vi "rewindDir_printDirectory.vi"(8 "Error In":errorcluster, 10 "nested level":u8, 11 "file":refnum<class "File.lvclass">) -> (0 "Error Out":errorcluster)   [LabVIEW 2014, in "LabVIEW Universal Transcriptor SD Card Library.lvlib"]
uses:
  LabVIEW Universal Transcriptor SD Card Library.lvlib
  File.lvclass
  File.lvclass/File.ctl
  File Class/Get If Rewind This Directory.vi
  <vilib>/Utility/file.llb/Application Directory.vi
  open.vi
  <vilib>/LabVIEW Universal Transcriptor/LabVIEW to Arduino Transcriptor/Transcriptors/System API/Serial println string.vi
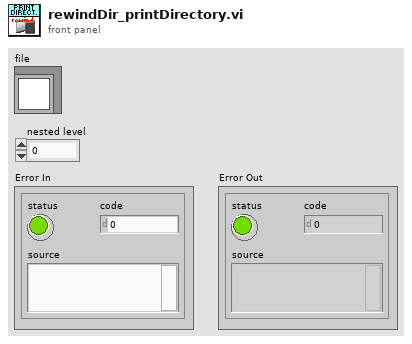
[diagram p1: front panel]
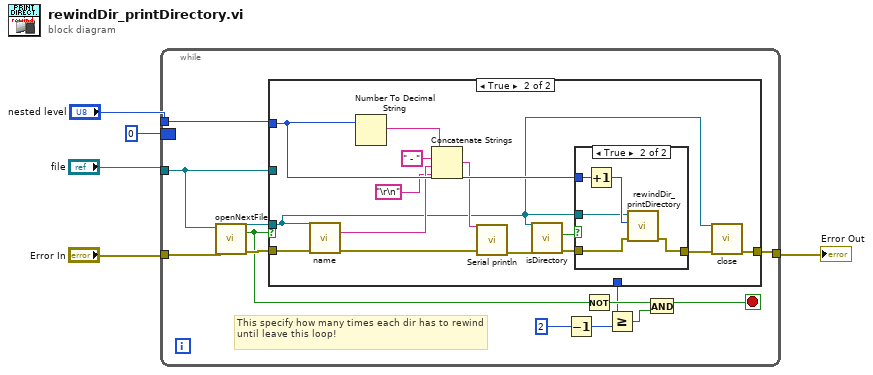
[diagram p0: block diagram]
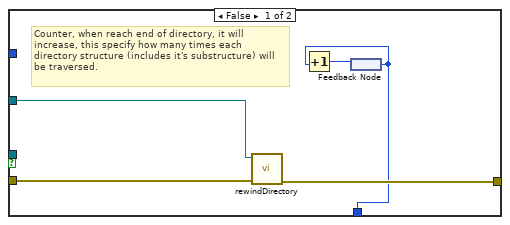
[diagram p2: hidden frame]
diagram:
  n1 = while {
    tunnel: "nested level" -> [w15]
    tunnel: "Error In" -> [w9]
    tunnel: [w16] -> w2
    tunnel: "file" -> [w8]
    border: 0 ("y") -> [_]
    stop <- w12 stop-if-true
    # "This specify how many times each dir has to rewind until leave this loop!"
    n2 = call "openNextFile.vi"("error in (no error)"=w9, "File in"=w8) -> ("error out"=w17:errorcluster, "success?"=w13:bool, "File out"=w18:refnum<class "File.lvclass">)  [unwired: 7 in]
    n3 = case shown="True" w13 {
      tunnel: w18 -> [_ w26]
      tunnel: w17 -> [w23 w37]
      tunnel: [w22 w28] -> w16
      tunnel: w15 -> [_ w33]
      tunnel: w8 -> [w21 _]
      tunnel: [w19 _] -> w7
      frame False {
        # "Counter, when reach end of directory, it will increase, this specify how many times each directory structure (includes it's substructure) will be traversed."
        n4 = call-dynamic "rewindDirectory.vi"("error in (no error)"=w23, "File in"=w21) -> ("error out"=w22:errorcluster)  [unwired: 9 in]
        n5 = feedback #1() -> (w19:i32)
        n6 = Increment(x=w19) -> (x+1=w20:i32)
        n7 = feedback-in #1(w20) -> ()
      }
      frame True {
        n8 = call-dynamic "name.vi"("error in (no error)"=w37, "File in"=w26) -> ("error out"=w36:errorcluster, "file name"=w27:string)  [unwired: 8 in]
        n9 = Number To Decimal String(number=w33) -> (decimal integer string=w32:string)  [unwired: 1 in]
        n10 = Concatenate Strings(w32, " - " ("string"), w27, "\r\n") -> (w30:string)
        n11 = call-poly <vilib>:"Serial println.vi"("Error In"=w36, "string in"=w30) -> ("Error Out"=w35:errorcluster)  [unwired: 9 in]
        n12 = call-dynamic "isDirectory.vi"("error in (no error)"=w35, "File in"=w26) -> ("error out"=w34:errorcluster, "is directory?"=w25:bool)  [unwired: 8 in]
        n13 = case shown="True" w25 {
          tunnel: w34 -> [w38 w42]
          tunnel: [w38 w41] -> w29
          tunnel: w26 -> [_ w39]
          tunnel: w33 -> [_ w43]
          frame False {
          }
          frame True {
            n14 = Increment(x=w43) -> (x+1=w40:u8)
            n15 = call "rewindDir_printDirectory.vi"("Error In"=w42, "nested level"=w40, "file"=w39) -> ("Error Out"=w41:errorcluster)  [unwired: 8 in]
          }
        }
        n16 = call-dynamic "close.vi"("error in (no error)"=w29, "File in"=w26) -> ("error out"=w28:errorcluster)  [unwired: 9 in]
      }
    }
    n17 = Decrement(x=2 ("y")) -> (x-1=w6:i32)
    n18 = Not(x=w13) -> (.not. x?=w14:bool)
    n19 = Greater Or Equal?(x=w7, y=w6) -> (x >= y?=w11:bool)
    n20 = And(x=w14, y=w11) -> (x .and. y?=w12:bool)
  }
  "Error Out" <- w2
